vi "Msg.vi"(7 "Actor in":refnum<class "Actor.lvclass">, 11 "Update Pump State Msg in":refnum<class "Update Pump State Msg.lvclass">) -> (0 "Error out":errorcluster, 5 "Actor out":refnum<class "Actor.lvclass">)   [LabVIEW 2025, in "Update Pump State Msg.lvlib" / "Update Pump State Msg.lvclass"]
uses:
  Update Pump State Msg.lvclass
  <vilib>/Nathan Davis/jettl/jettl/jettl/Actor/Actor/Actor.lvclass
  Update Pump State/Update Pump State.lvclass
  Update Pump State Msg.lvclass/Update Pump State Msg.ctl
panel:
  # "This front panel should not be manipulated."
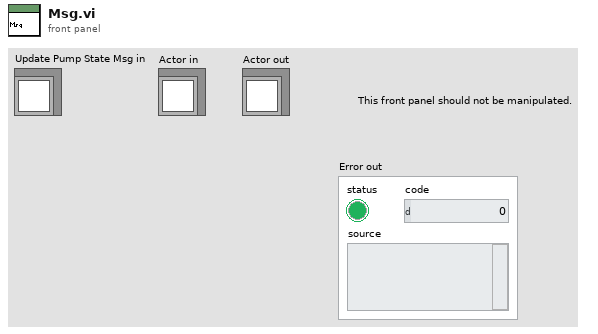
[diagram p1: front panel]
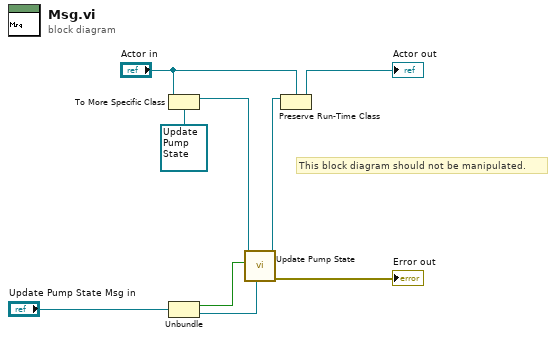
[diagram p0: block diagram]
diagram:
  # "This block diagram should not be manipulated."
  n1 = To More Specific Class(target class=refnum<class "Update Pump State.lvclass"> refnum ("jettl Msg Template"), reference="Actor in") -> (specific class reference=w7:refnum<class "Update Pump State.lvclass">)  [unwired: 1 in, 1 out]
  n2 = Unbundle "Unbundle"("Update Pump State Msg in") -> (w2:bool, w1:refnum<class "Sender.lvclass">)
  n3 = call-dynamic "Update Pump State.vi"("Sender"=w1, "Pump State"=w2, "Update Pump State in"=w7) -> ("Error out"=→"Error out":errorcluster, "Update Pump State out"=w6:refnum<class "Update Pump State.lvclass">)  [unwired: 7 in]
  n4 = Preserve Run-Time Class(object in=w6, 2:"Actor in") -> (object out=→"Actor out":refnum<class "Actor.lvclass">)  [unwired: 1 in, 1 out]
